vi "Clase8.vi"() -> ()   [LabVIEW 2013]
panel:
  out "potencia":dbl
  out "exponente":dbl
  out "base":dbl
  # "Generar la base y el exponente con numeros del 1-10\nluego generar la potencia usando ciclo for"
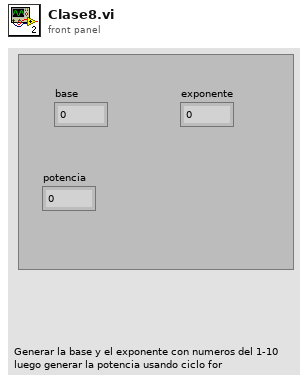
[diagram p1: front panel]
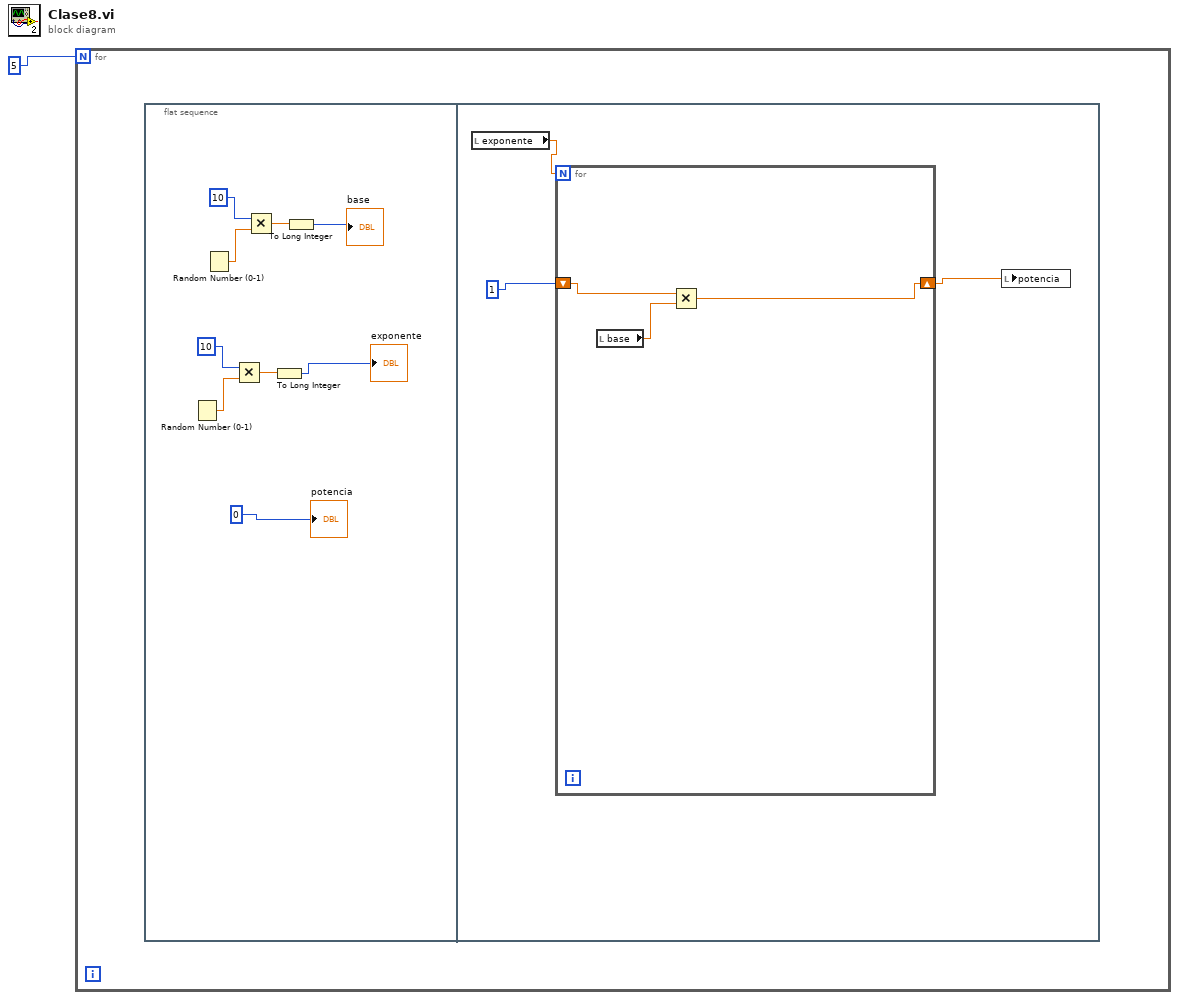
[diagram p0: block diagram]
diagram:
  n1 = for {
    N: 5 -> [_]
    n2 = flat-sequence {
      frame #0 {
        n3 = Random Number (0-1)() -> (number: 0 to 1=w5:dbl)
        n4 = Random Number (0-1)() -> (number: 0 to 1=w9:dbl)
        n5 = Multiply(x=10, y=w5) -> (x*y=w6:dbl)
        n6 = Multiply(x=10, y=w9) -> (x*y=w8:dbl)
        n7 = To Long Integer(number=w6) -> (32bit integer=→"exponente":i32)
        n8 = To Long Integer(number=w8) -> (32bit integer=→"base":i32)
        "potencia" <- 0
      }
      frame #1 {
        n9 = local read "exponente"() -> (w13:dbl)
        n10 = for {
          N: w13 -> [_]
          shift-right: [w14] -> w11
          shift-left: 1 -> [w16]
          n11 = local read "base"() -> (w15:dbl)
          n12 = Multiply(x=w16, y=w15) -> (x*y=w14:dbl)
        }
        n13 = local write "potencia"(w11) -> ()
      }
    }
  }
